vi "Test Report Path Is Used on Open.vi"(8 "error in (no error)":errorcluster, 11 "XML Report Test in":refnum<class "Report Generator Test.lvclass">) -> (0 "error out":errorcluster, 3 "XML Report Test out":refnum<class "Report Generator Test.lvclass">)   [LabVIEW 2020, in "Report Generator Test.lvclass"]
uses:
  Report Generator Test.lvclass
  C:/Program Files (x86)/National Instruments/LabVIEW 2020/vi.lib/Astemes/LUnit/Test Case.lvclass
  <vilib>/Astemes/LUnit/Test Case.lvclass/Test Case.ctl
  bd454a0f-0b48-4323-aa23-a3078375362f.vi
  <vilib>/Astemes/LUnit/Palette/Pass.vi
  <vilib>/Astemes/LUnit/Palette/Fail.vi
  <vilib>/Astemes/LUnit/Compare Variants.vi
  <vilib>/Astemes/LUnit/Describe Comparison.vi
  <vilib>/Astemes/LUnit/Set Assertion Type.vi
  <vilib>/Astemes/LUnit/Add test result.vi
  <vilib>/Astemes/LUnit/Variant to string.vi
  <vilib>/Astemes/LUnit/LUnit Record Assertion Result.vi
  <vilib>/Astemes/LUnit/LUnit Aggregate Assertion Results.vi
  <vilib>/Astemes/LUnit/Method Result/LUnit Merge Status.vi
  <vilib>/Astemes/LUnit/LUnit Concatenate result strings.vi
  Test Doubles/Mock Report/Mock Report.lvclass
  C:/git/astemes-lunit/source/Plugins/Report/Report.lvclass
  <vilib>/Utility/Data Type/Get Type Information.vi
  <vilib>/Utility/LVClass/Get LV Class Name.vi
  Report Generator Test.lvclass/Report Generator Test.ctl
  source/Plugins/Report/Report.lvclass
  C:/git/astemes-lunit/source/Plugins/Plugin/Plugin.lvclass
  C:/git/astemes-lunit/source/Framework/Result Observer/Result Observer.lvclass
  C:/git/astemes-lunit/source/Plugins/Report Interface/Report Interface.lvclass
  C:/git/astemes-lunit/tests/Test Doubles/Mock Report/Mock Report.lvclass
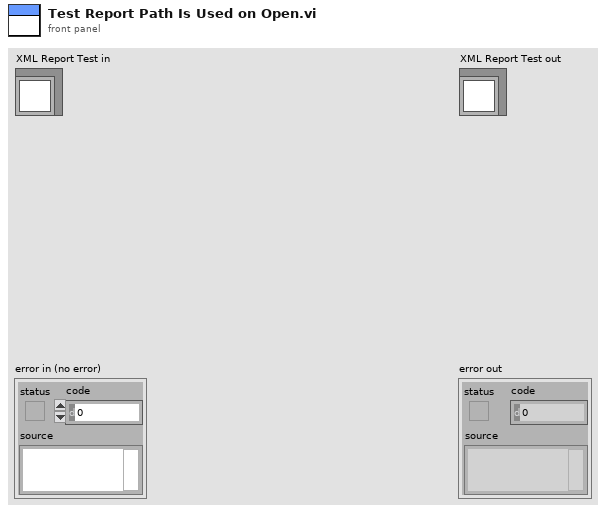
[diagram p1: front panel]
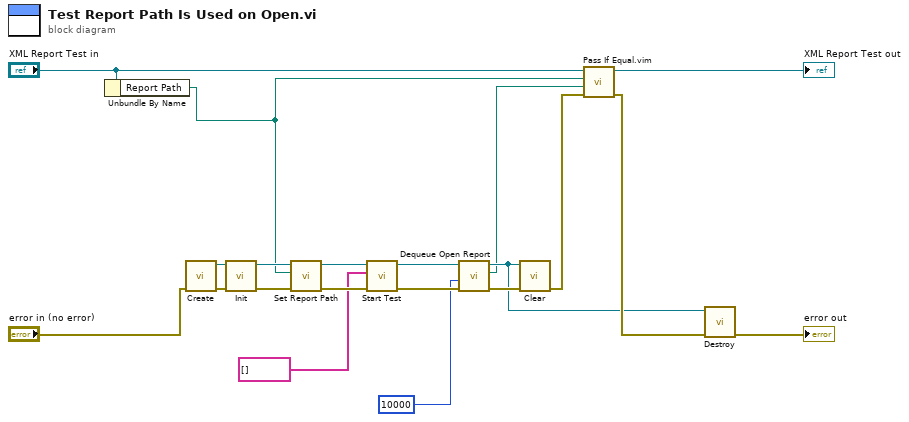
[diagram p0: block diagram]
diagram:
  n1 = Unbundle By Name("XML Report Test in") -> ("Report Path"=w1:path)
  n2 = call "Create.vi"("error in (no error)"="error in (no error)") -> ("error out"=w12:errorcluster, "Mock Report Out"=w4:refnum<class "Mock Report.lvclass">)  [unwired: 9 in]
  n3 = call-dynamic "Init.vi"("error in (no error)"=w12, "Mock Report In"=w4) -> ("error out"=w5:errorcluster, "Mock Report Out"=w3:refnum<class "Mock Report.lvclass">)  [unwired: 8 in]
  n4 = call "Set Report Path.vi"("error in (no error)"=w5, "Report Path"=w1, "Report In"=w3) -> ("error out"=w17:errorcluster, "Report Out"=w18:refnum<class "Mock Report.lvclass">)  [unwired: 7 in]
  n5 = call-dynamic "Start Test.vi"("error in (no error)"=w17, "Tests"=string[] [], "XML Report in"=w18) -> ("error out"=w16:errorcluster, "XML Report out"=w15:refnum<class "Mock Report.lvclass">)  [unwired: 7 in]
  n6 = call "Dequeue Open Report.vi"("error in (no error)"=w16, "timeout in ms (0)"=10000, "Mock Report In"=w15) -> ("error out"=w14:errorcluster, "path"=w7:path, "Mock Report Out"=w10:refnum<class "Mock Report.lvclass">)  [unwired: 5 in, 1 out]
  n7 = call-dynamic "Clear.vi"("error in (no error)"=w14, "XML Report in"=w10) -> ("error out"=w6:errorcluster)  [unwired: 9 in]
  n8 = call "Pass If Equal.vim"("error in (no error)"=w6, "Actual"=w7, "Expected"=w1, "LUnit Test Case In"="XML Report Test in") -> ("error out"=w19:errorcluster, "LUnit Test Case Out"=→"XML Report Test out":refnum<class "Report Generator Test.lvclass">)  [unwired: 6 in]
  n9 = call "Destroy.vi"("error in (no error)"=w19, "Mock Report In"=w10) -> ("error out"=→"error out":errorcluster)  [unwired: 9 in]
